vi "Format Number with SD.vi"(9 "Number of readings in Mean":i32, 10 "SD":dbl, 11 "Mean":dbl) -> (2 "Formated SD":string, 3 "Formated Mean":string)   [LabVIEW 2020, in "Library Commun.lvlib" / "JSON Statistics.lvclass"]
uses:
  JSON Statistics.lvclass
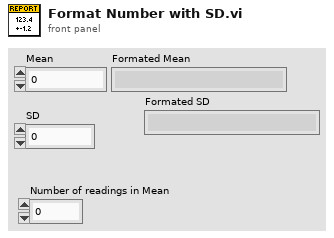
[diagram p1: front panel]
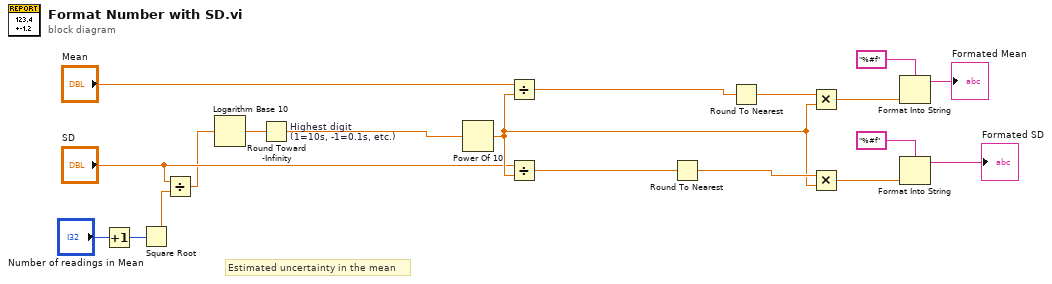
[diagram p0: block diagram]
diagram:
  # "Estimated uncertainty in the mean"
  n1 = Increment(x="Number of readings in Mean") -> (x+1=w5:i32)
  n2 = Square Root(x=w5) -> (sqrt(x)=w3:dbl)
  n3 = Divide(x="SD", y=w3) -> (x/y=w2:dbl)
  n4 = Logarithm Base 10(1:w2) -> (0:w19:dbl)
  n5 = Round Toward -Infinity "Highest digit\n(1=10s, -1=0.1s, etc.)"(1:w19) -> (0:w1:dbl)
  n6 = Power Of 10(x=w1) -> (10^x=w7:dbl)
  n7 = Divide(x="Mean", y=w7) -> (x/y=w12:dbl)
  n8 = Divide(x="SD", y=w7) -> (x/y=w13:dbl)
  n9 = Round To Nearest(number=w13) -> (nearest integer value=w16:dbl)
  n10 = Round To Nearest(number=w12) -> (nearest integer value=w11:dbl)
  n11 = Multiply(x=w11, y=w7) -> (x*y=w10:dbl)
  n12 = Multiply(x=w16, y=w7) -> (x*y=w15:dbl)
  n13 = Format Into String(format string="%#f", w10) -> (resulting string=→"Formated Mean":string)  [unwired: 2 in, 1 out]
  n14 = Format Into String(format string="%#f", w15) -> (resulting string=→"Formated SD":string)  [unwired: 2 in, 1 out]
